vi "Get PDO Mappables.vi"(8 "error in":errorcluster, 10 "Type":enum16{"RX", "TX"}(ring), 11 "Object Dictionary in":refnum<class "Object Dictionary.lvclass">) -> (0 "error out":errorcluster, 2 "PDO Mappables":T2(array[cluster]) {"Data Type" items=["unknown", "BOOLEAN", "INTEGER8", "INTEGER16", "INTEGER32", "UNSIGNED8", "UNSIGNED16", "UNSIGNED32", "REAL32", "VISIBLE_STRING", "OCTET_STRING", "UNICODE_STRING", "TIME_OF_DAY", "TIME_DIFFERENCE", "RESERVED1", "DOMAIN", "INTEGER24", "REAL64", "INTEGER40", "INTEGER48", "INTEGER56", "INTEGER64", "UNSIGNED24", "RESERVED2", "UNSIGNED40", "UNSIGNED48", "UNSIGNED56", "UNSIGNED64", "RESERVED3", "RESERVED4", "RESERVED5", "RESERVED6", "PDO_COMMUNICATION_PARAMETER", "PDO_MAPPING", "SDO_PARAMETER", "IDENTITY", "RESERVED7"]; "Index" format="%04x"; "Sub Index" format="%02x"}, 3 "Object Dictionary out":refnum<class "Object Dictionary.lvclass">)   [LabVIEW 2020, in "CANopen.lvlib"]
uses:
  CANopen.lvlib
  Object Dictionary/Object Dictionary.lvclass
  Sub Object/Sub Object.lvclass/Sub Object.ctl
  Sub Object/Sub Object.lvclass
  Typedefs/Data Type.ctl
  Object Entry/Object Entry.lvclass
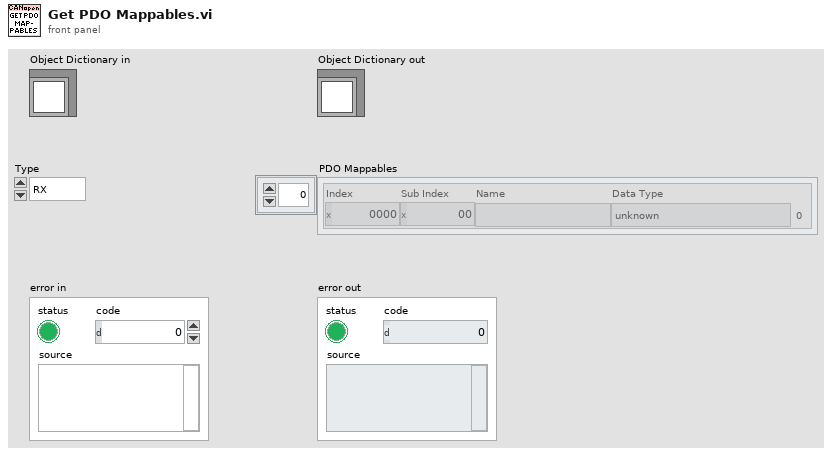
[diagram p1: front panel]
types:
  T1 = typedef "CANopen.lvlib/Data Type.ctl" = u16
  T2 = cluster{"Index":u16, "Sub Index":u8, "Name":string, "Data Type":T1}[]
  T3 = cluster{"Index":u16, "Sub Index":u8, "Name":string, "Data Type":T1}
  T4 = typedef "CANopen.lvlib/Access Type.ctl" = enum16{"unknown", "ro", "wo", "rw", "rwr", "rww", "const"}
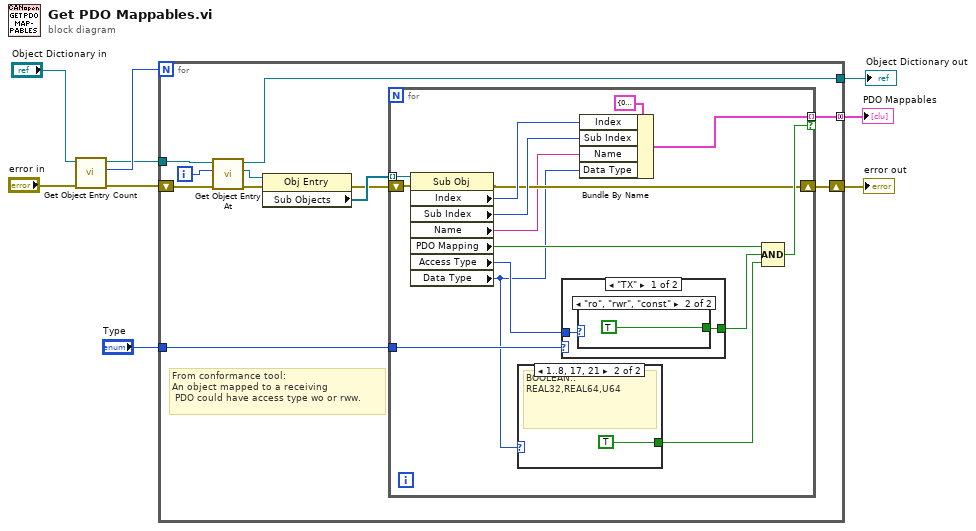
[diagram p0: block diagram]
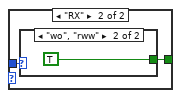
[diagram p3: hidden frame]
diagram:
  n1 = call "Get Object Entry Count.vi"("error in"="error in", "Obj Dict in"="Object Dictionary in") -> ("error out"=w5:errorcluster, "Count"=w7:i32, "Obj Dict out"=w6:refnum<class "Object Dictionary.lvclass">)  [unwired: 7 in]
  n2 = for {
    N: w7 -> [_]
    tunnel: w6 -> [w19]
    tunnel: [w13] -> w3 mode=concatenating
    shift-right: [w12] -> w4
    shift-left: w5 -> [w20]
    tunnel: [w11] -> w2
    tunnel: "Type" -> [w10]
    i -> [w18]
    # "From conformance tool:\nAn object mapped to a receiving\n PDO could have access type wo or rww."
    n3 = call "Get Object Entry At.vi"("error in"=w20, "Index"=w18, "Obj Dict in"=w19) -> ("error out"=w17:errorcluster, "Obj Entry"=w16:refnum<class "Object Entry.lvclass">, "Obj Dict out"=w11:refnum<class "Object Dictionary.lvclass">)  [unwired: 6 in]
    n4 = property class="Obj Entry"(reference=w16, error in=w17) -> (error out=w14:errorcluster, "Sub Objects"=w15:refnum<class "Sub Object.lvclass">[])  [unwired: 1 out]
    n5 = for {
      tunnel: w15 -> [w34] mode=indexing
      tunnel: [w29] -> w13 mode=indexing if=w28
      shift-right: [w27] -> w12
      shift-left: w14 -> [w35]
      tunnel: w10 -> [w22]
      n6 = property class="Sub Obj"(reference=w34, error in=w35) -> (error out=w27:errorcluster, "Index"=w32:u16, "Sub Index"=w31:u8, "Name"=w26:string, "PDO Mapping"=w33:bool, "Access Type"=w25:T4, "Data Type"=w21:T1)  [unwired: 1 out]
      n7 = case shown="1..8, 17, 21" w21 {
        tunnel: [_ TRUE] -> w23
        frame 0, Default {
        }
        frame 1..8, 17, 21 {
          # "BOOLEAN..REAL32,REAL64,U64"
        }
      }
      n8 = case shown="\"TX\"" w22 {
        tunnel: w25 -> [w37 w40]
        tunnel: [w36 w39] -> w24
        frame "TX" {
          n9 = case shown="\"ro\", \"rwr\", \"const\"" w37 {
            tunnel: [_ TRUE] -> w36
            frame "unknown", Default {
            }
            frame "ro", "rwr", "const" {
            }
          }
        }
        frame "RX" {
          n10 = case shown="\"wo\", \"rww\"" w40 {
            tunnel: [_ TRUE] -> w39
            frame "unknown", Default {
            }
            frame "wo", "rww" {
            }
          }
        }
      }
      n11 = Bundle By Name(cluster=T3 {"Index"=0, "Sub Index"=0, "Name"="", "Data Type"=0}, "Index"=w32, "Sub Index"=w31, "Name"=w26, "Data Type"=w21) -> (w29:T3)
      n12 = Compound Arithmetic op=AND(w33, w24, w23) -> (w28:bool)
    }
  }
  "Object Dictionary out" <- w2
  "error out" <- w4
  "PDO Mappables" <- w3
